vi "20211008_00.vi"() -> ()   [LabVIEW 2019]
panel:
  out "Num Array Max to Min":dbl[](array[numeric])
  out "Num Array < Avg.":dbl[](array[numeric])
  out "Num Array > Avg.":dbl[](array[numeric])
  out "Array Min":dbl
  out "Array Max":dbl
  out "Array Avg.":dbl
  in  "Num Array":dbl[](array[numeric])
  in  "N4":dbl
  in  "N3":dbl
  in  "N2":dbl
  in  "N1":dbl
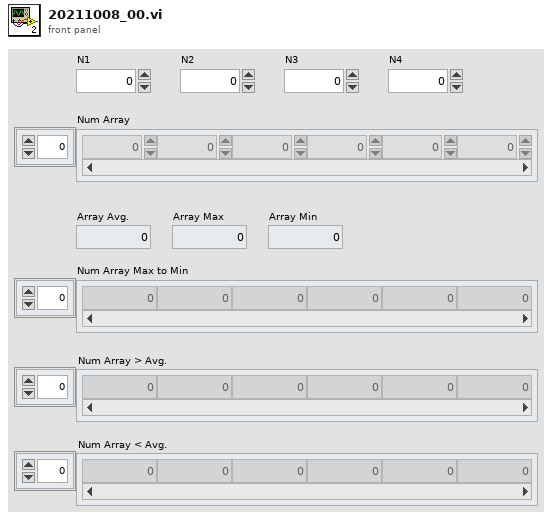
[diagram p1: front panel]
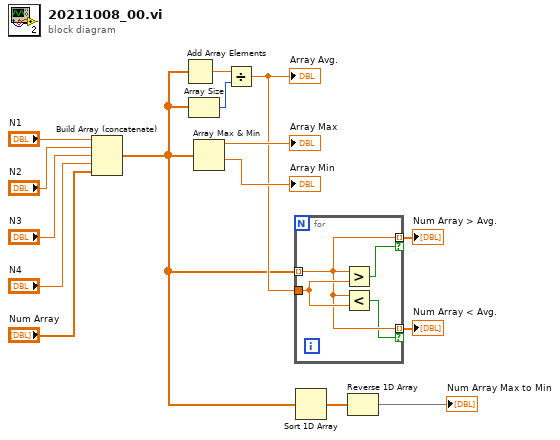
[diagram p0: block diagram]
diagram:
  n1 = Build Array (concatenate)("N1", "N2", "N3", "N4", "Num Array") -> (w1:dbl[])
  n2 = Add Array Elements(numeric array=w1) -> (sum=w10:dbl)
  n3 = Array Size(array=w1) -> (size(s)=w9:i32)
  n4 = Array Max & Min(array=w1) -> (max value=→"Array Max":dbl, min value=→"Array Min":dbl)  [unwired: 2 out]
  n5 = Divide(x=w10, y=w9) -> (x/y=w4:dbl)
  "Array Avg." <- w4
  n6 = for {
    tunnel: w1 -> [w17] mode=indexing
    tunnel: w4 -> [w19]
    tunnel: [w17] -> w6 mode=indexing if=w18
    tunnel: [w17] -> w5 mode=indexing if=w16
    n7 = Greater?(x=w17, y=w19) -> (0:w18:bool)
    n8 = Less?(x=w17, y=w19) -> (x < y?=w16:bool)
  }
  "Num Array > Avg." <- w6
  "Num Array < Avg." <- w5
  n9 = Sort 1D Array(array=w1) -> (sorted array=w3:dbl[])
  n10 = Reverse 1D Array(array=w3) -> (reversed array=→"Num Array Max to Min":dbl[])
